vi "Read.vi"(8 "error in (no error)":errorcluster, 11 "Add in":refnum<class "AbsFunc_One Term_U16.lvclass">) -> (0 "error out":errorcluster, 2 "Numeric":T1, 3 "Add out":refnum<class "AbsFunc_One Term_U16.lvclass">)   [LabVIEW 2021, in "AbsFunc_One Term_U16.lvclass"]
uses:
  AbsFunc_One Term_U16.lvclass
  Support/Data Type.ctl
  AbsFunc_One Term_U16.lvclass/AbsFunc_One Term_U16.ctl
  Abs_Types/U16 Integer/Abs_U16 Integer.lvclass
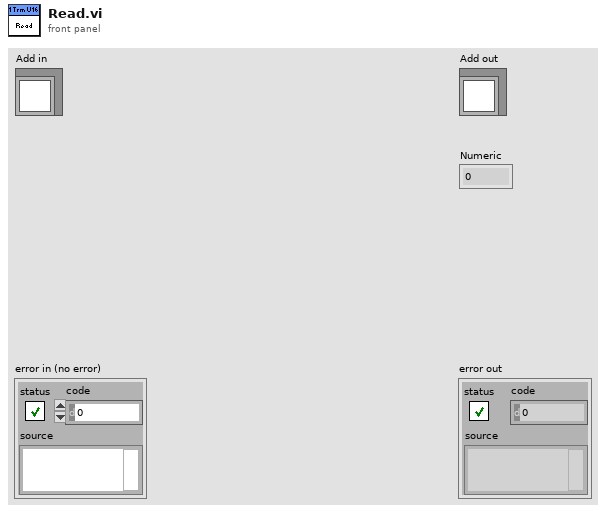
[diagram p1: front panel]
types:
  T1 = typedef "AbsFunc_One Term_U16.lvclass/Data Type.ctl" = u16
  T2 = typedef "AbsFunc_One Term_U16.lvclass/Abstract Type.ctl" = refnum<class "Abs_U16 Integer.lvclass">
  T3 = typedef "Abs_U16 Integer.lvclass/Type.ctl" = u16
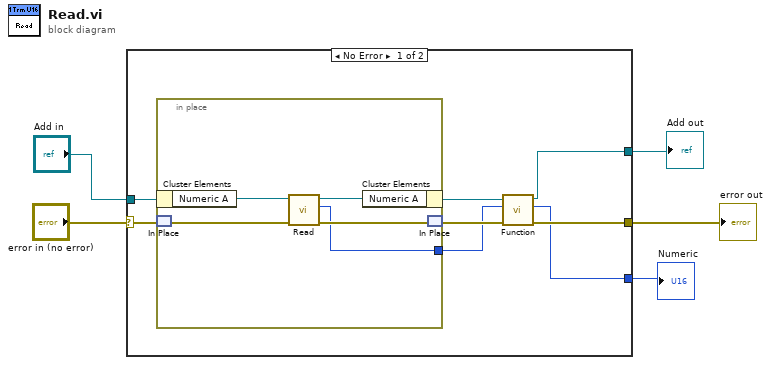
[diagram p0: block diagram]
diagram:
  n1 = case shown="No Error" "error in (no error)" {
    selector: "error in (no error)" -> [w12 w19]
    tunnel: "Add in" -> [w13 w20]
    tunnel: [w9 w20] -> w3
    tunnel: [w8 w19] -> w2
    tunnel: [w6 _] -> w1
    frame No Error {
      n2 = in-place {
        in-place-border: [w14] -> w7
        n3 = in-place-cluster #1(w13) -> ("Numeric A"=w18:T2)
        n4 = in-place-match #2(w12) -> (w16:errorcluster)
        n5 = call-dynamic "Read.vi"("error in (no error)"=w16, "Double Float.lvclass_340760 in"=w18) -> ("error out"=w15:errorcluster, "Value"=w14:T3, "Double Float.lvclass_340760 out"=w17:T2)  [unwired: 7 in]
        n6 = in-place-cluster #1("Numeric A"=w17) -> (w10:refnum<class "AbsFunc_One Term_U16.lvclass">)
        n7 = in-place-match #2(w15) -> (w11:errorcluster)
      }
      n8 = call-dynamic "Function.vi"("error in (no error)"=w11, "Numeric A"=w7, "Two Terminal in"=w10) -> ("error out"=w8:errorcluster, "Result"=w6:T1, "Two Terminal out"=w9:refnum<class "AbsFunc_One Term_U16.lvclass">)  [unwired: 6 in]
    }
    frame Error {
    }
  }
  "error out" <- w2
  "Add out" <- w3
  "Numeric" <- w1
